vi "MLEfitPicture.vi"(2 "threshold":u32, 3 "plane":i32, 4 "channel":u8=1, 5 "F2-channel":u8) -> (0 "Lifetimes":dbl[][](array[numeric]) format="%.2f", 1 "F2-values":sgl[][](array[numeric]) format="%.2f")   [LabVIEW 2009]
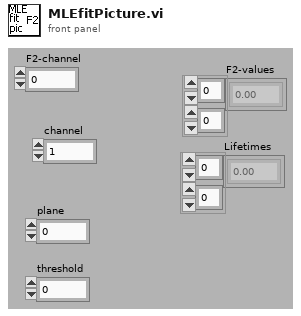
[diagram p1: front panel]
types:
  T1 = enum16{"Display", "change", "Get", "Set", "Set Ken"}
  T2 = typedef "FIFOSettings_BH.ctt" = cluster{"Measurement":cluster{"Binning (ms)":sgl, "External Trigger Condition":u16, "Stop Condition:":u16, "Stop Count":dbl, "Buffer Size (Photons)":u16, "No of Channels":u16, "Ext Latch Delay":i16}, "ADC":cluster{"Module":u16, "ADC Resolution":i32, "Dither Range":i16, "Count Increment":i16, "Macro Time Clock":i16}, "SYNC":cluster{"SYNC ZC Level (mV)":sgl, "SYNC Freq Divider":i16, "SYNC Holdoff (ns)":sgl, "SYNC Threshold (mV)":sgl}, "TAC":cluster{"TAC Range (ns)":sgl, "TAC Gain":i16, "TAC Offset (%)":sgl, "TAC Limit Low (%)":sgl, "TAC Limit High (%)":sgl}, "CFD":cluster{"CFD Limit Low (mV)":sgl, "CFD Limit High (mV)":sgl, "CFD ZC Level (mV)":sgl, "CFD Holdoff (ns)":sgl}}
  T3 = typedef "Settings.ctl" = cluster{"threshold":cluster{"max":u32, "min":u32}, "RGB or false color":bool, "16bit":bool, "log/lin axis":u16, "spotsize button":bool, "Pixelsize":u16, "autoscale x":bool, "autoscale y":bool, "correlation":bool, "ADC-Resolution":i32, "F2-lifetime":cluster{"display tau":bool, "display F2":bool, "Palette Number lifetime":enum32{"Gray", "Binary", "Gradient", "Rainbow", "Temperature"}, "Palette Number F2":enum32{"Gray", "Binary", "Gradient", "Rainbow", "Temperature"}, "max tau-Value":dbl, "min tau-Value":dbl, "max F2-Value":dbl, "min F2-Value":dbl}, "TAC-Window 1":u16, "TAC-Window 2":u16, "false color palette":cluster{"1":u32, "2":u32, "3":u32, "4":u32, "5":u32, "6":u32, "7":u32, "8":u32, "8 2":u32, "8 3":u32, "8 4":u32, "8 5":u32}}
  T4 = cluster{"router":u8[], "macro times":dbl[], "micro times":u16[], "invalid":dbl[], "gap":dbl[]}
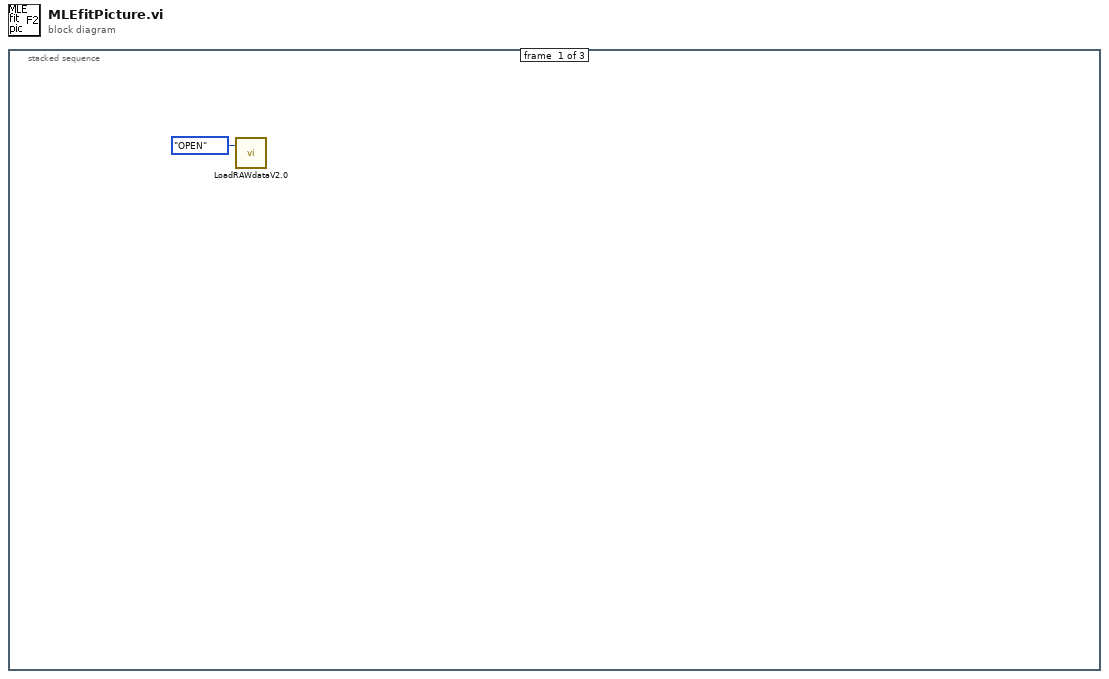
[diagram p0: block diagram]
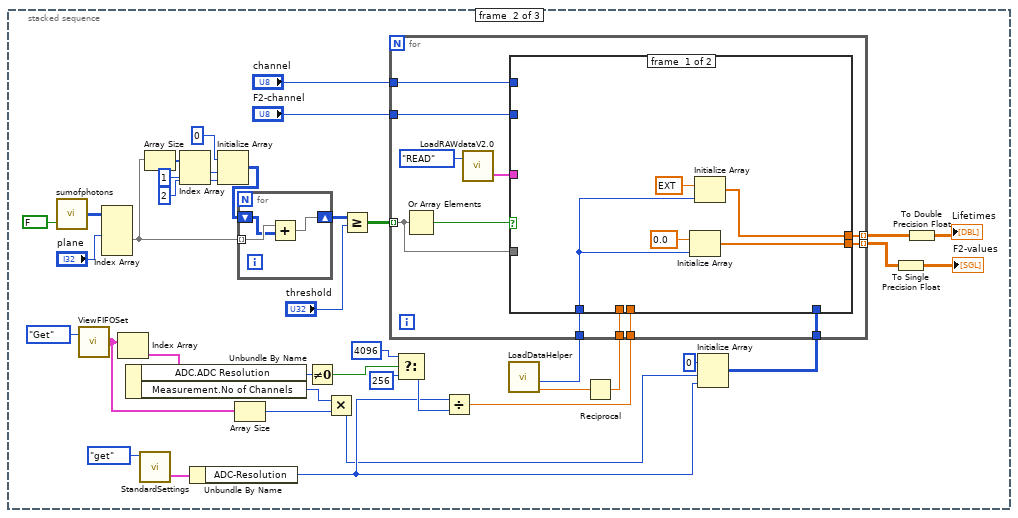
[diagram p2: hidden frame]
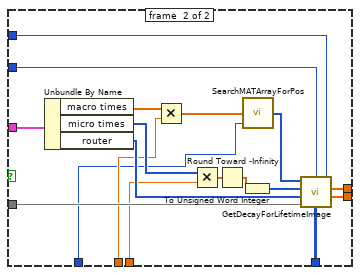
[diagram p3: hidden frame]
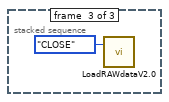
[diagram p4: hidden frame]
diagram:
  n1 = stacked-sequence {
    frame #0 {
      n2 = call "LoadRAWdataV2.0.vi"("action"=enum16{"OPEN", "READ", "CLOSE"}."OPEN" ("Enum")) -> ()  [unwired: 1 in, 2 out]
    }
    frame #1 {
      n3 = call "sumofphotons.vi"("s"=FALSE) -> ("sum of photons out"=w40:u32[][][][])  [unwired: 1 in]
      n4 = call "ViewFIFOSet.vi"("Enum"=T1."Get") -> ("FIFO Settings (Array)"=w14:T2[])  [unwired: 1 in]
      n5 = Index Array(array=w40, index (dim 1)="plane") -> (element=w9:u32[][][])  [unwired: 3 in]
      n6 = Index Array(array=w14) -> (element=w15:T2)  [unwired: 1 in]
      n7 = Unbundle By Name(w15) -> ("ADC.ADC Resolution"=w31:i32, "Measurement.No of Channels"=w12:u16)
      n8 = call "StandardSettings.vi"("Enum"=enum16{"Load", "get", "Save", "set"}."get") -> ("StandardSettings"=w34:T3)  [unwired: 4 in]
      n9 = Array Size(array=w9) -> (size(s)=w8:i32[])
      n10 = Index Array(array=w8, index #1=1 ("index"), index #2=2 ("index")) -> (element #1=w5:i32, element #2=w4:i32)
      n11 = Unbundle By Name(w34) -> ("ADC-Resolution"=w17:i32)
      n12 = Initialize Array(0 ("element"), w5, w4) -> (w2:i32[][])
      n13 = Array Size(array=w14) -> (size(s)=w11:i32)
      n14 = for {
        tunnel: w9 -> [w78] mode=indexing
        shift-right: [w79] -> w37
        shift-left: w2 -> [w77]
        n15 = Add(x=w78, y=w77) -> (x+y=w79:u32[][])
      }
      n16 = Not Equal To 0?(x=w31) -> (x != 0?=w30:bool)
      n17 = Multiply(x=w12, y=w11) -> (x*y=w13:i32)
      n18 = Greater Or Equal?(x=w37, y="threshold") -> (x >= y?=w38:bool[][])
      n19 = Select(t=4096, s=w30, f=256) -> (s? t:f=w27:i32)
      n20 = Divide(x=w17, y=w27) -> (x/y=w26:dbl)
      n21 = call "LoadDataHelper.vi"() -> ("Time Resolution [ms/pixel]"=w10:dbl, "pixel per line"=w25:u32)  [unwired: 7 in, 3 out]
      n22 = Reciprocal(x=w10) -> (1/x=w20:dbl)
      n23 = Initialize Array(u32 0 ("element"), w13, w17) -> (w18:u32[][])
      n24 = for {
        tunnel: w38 -> [w52] mode=indexing
        tunnel: "F2-channel" -> [w51]
        tunnel: w26 -> [w50]
        tunnel: [w49] -> w24 mode=indexing
        tunnel: [w48] -> w23 mode=indexing
        tunnel: w25 -> [w47]
        tunnel: w20 -> [w46]
        tunnel: w18 -> [w45]
        tunnel: "channel" -> [w44]
        n25 = Or Array Elements(Boolean array=w52) -> (logical OR=w53:bool)
        n26 = call "LoadRAWdataV2.0.vi"("action"=enum16{"OPEN", "READ", "CLOSE"}."READ" ("Enum")) -> ("RAW data"=w43:T4)  [unwired: 1 in, 1 out]
        n27 = case shown="True" w53 {
          tunnel: w52 -> [_ w75]
          tunnel: w51 -> [_ w73]
          tunnel: w50 -> [_ w71]
          tunnel: [w56 w67] -> w49
          tunnel: [w55 w66] -> w48
          tunnel: w47 -> [w54 w63]
          tunnel: w46 -> [_ w64]
          tunnel: w45 -> [_ w62]
          tunnel: w44 -> [_ w61]
          tunnel: w43 -> [_ w60]
          frame #0 {
            n28 = Initialize Array(0.0 ("fit tau"), w54) -> (w55:dbl[])
            n29 = Initialize Array(ext 0.0 ("fit tau"), w54) -> (w56:ext[])
          }
          frame #1 {
            n30 = Unbundle By Name(w60) -> ("macro times"=w65:dbl[], "micro times"=w72:u16[], "router"=w74:u8[])
            n31 = Multiply(x=w65, y=w64) -> (x*y=w59:dbl[])
            n32 = Multiply(x=w72, y=w71) -> (x*y=w70:dbl[])
            n33 = Round Toward -Infinity(1:w70) -> (0:w69:dbl[])
            n34 = To Unsigned Word Integer(number=w69) -> (unsigned 16bit integer=w68:u16[])
            n35 = call "SearchMATArrayForPos.vi"("pixel per line"=w63, "macro times"=w59) -> ("Array"=w76:i32[])  [unwired: 3 in]
            n36 = call "GetDecayForLifetimeImage.vi"("channel"=w61, "F2-channel"=w73, "Array 2"=w76, "micro times"=w68, "empty decay"=w62, "router"=w74, "Array"=w75) -> ("lifetime [ns]"=w67:ext[], "F2-value"=w66:dbl[])  [unwired: 1 in]
          }
        }
      }
      n37 = To Single Precision Float(number=w23) -> (single precision float=→"F2-values":sgl[][])
      n38 = To Double Precision Float(number=w24) -> (double precision float=→"Lifetimes":dbl[][])
    }
    frame #2 {
      n39 = call "LoadRAWdataV2.0.vi"("action"=enum16{"OPEN", "READ", "CLOSE"}."CLOSE" ("Enum")) -> ()  [unwired: 1 in, 2 out]
    }
  }
